vi "Stop TS DAC.vi"(8 "error in (no error)":errorcluster, 11 "Generic Test Stand in":refnum<class "Generic Test Stand.lvclass">) -> (0 "error out":errorcluster, 3 "Generic Test Stand out":refnum<class "Generic Test Stand.lvclass">)   [LabVIEW 2019, in "Generic Test Stand.lvclass"]
uses:
  Generic Test Stand.lvclass
  Generic Test Stand.lvclass/Generic Test Stand.ctl
  DAC/DAC.lvclass
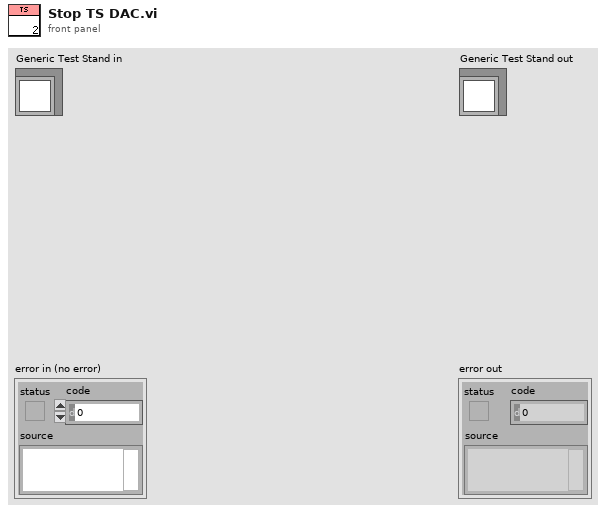
[diagram p1: front panel]
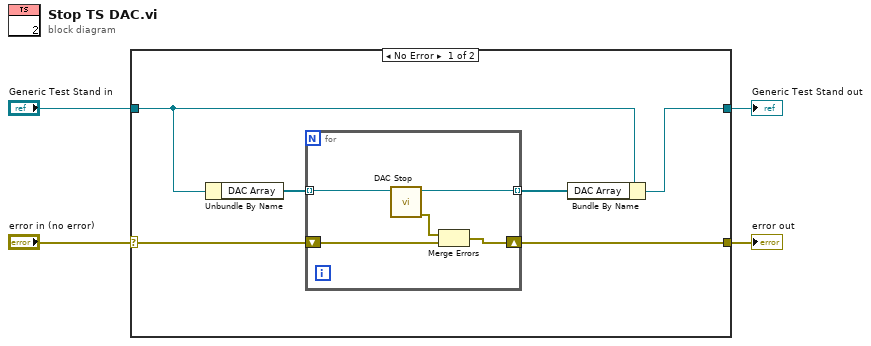
[diagram p0: block diagram]
diagram:
  n1 = case shown="No Error" "error in (no error)" {
    selector: "error in (no error)" -> [w9 w17]
    tunnel: [w5 w17] -> w3
    tunnel: [w6 w16] -> w1
    tunnel: "Generic Test Stand in" -> [w7 w16]
    frame No Error {
      n2 = Unbundle By Name(w7) -> ("DAC Array"=w10:refnum<class "DAC.lvclass">[])
      n3 = for {
        tunnel: w10 -> [w13] mode=indexing
        shift-right: [w14] -> w5
        shift-left: w9 -> [w15]
        tunnel: [w12] -> w8 mode=indexing
        n4 = call-dynamic "DAC Stop.vi"("DAC in"=w13) -> ("error out"=w11:errorcluster, "DAC out"=w12:refnum<class "DAC.lvclass">)  [unwired: 9 in]
        n5 = Merge Errors(w11, w15) -> (w14:errorcluster)
      }
      n6 = Bundle By Name(cluster=w7, "DAC Array"=w8) -> (w6:refnum<class "Generic Test Stand.lvclass">)
    }
    frame Error {
    }
  }
  "error out" <- w3
  "Generic Test Stand out" <- w1
